vi "Measure_CH3-4.vi"() -> ()   [LabVIEW 2018]
uses:
  Agilent N6700 Series/Agilent N6700 Series.lvlib
panel:
  in  "Measurement Type (1: Voltage)":i32(ring)=1 items=["Current", "Voltage", "Power"]
  out "CH4":dbl format="%^.3e"
  out "CH3":dbl format="%^.3e"
  in  "VISA resource name":refnum<visa-resource-name>
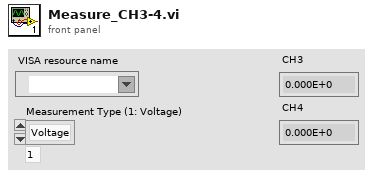
[diagram p1: front panel]
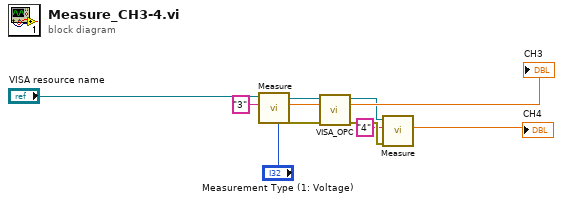
[diagram p0: block diagram]
diagram:
  n1 = call "Measure.vi"("Measurement Type (1: Voltage)"="Measurement Type (1: Voltage)", "Channel Name (1)"="3", "VISA resource name"="VISA resource name") -> ("error out"=w8:errorcluster, "Measurement"=→"CH3":dbl, "VISA resource name out"=w3:refnum<visa-resource-name>)  [unwired: 6 in]
  n2 = call "VISA_OPC.vi"("error in"=w8, "Session In"=w3) -> ("error out"=w5:errorcluster, "Session Out"=w4:refnum<visa-resource-name>)  [unwired: 7 in, 1 out]
  n3 = call "Measure.vi"("error in (no error)"=w5, "Channel Name (1)"="4", "VISA resource name"=w4) -> ("Measurement"=→"CH4":dbl)  [unwired: 6 in, 2 out]
